vi "Set Tilt Degree (SubVI).vi"(0 "handle in":i64, 1 "degree":i32, 3 "error in (no error)":errorcluster) -> (7 "handle out":i64, 10 "error out":errorcluster)   [LabVIEW 2017]
uses:
  libkinect_wrapper.dll
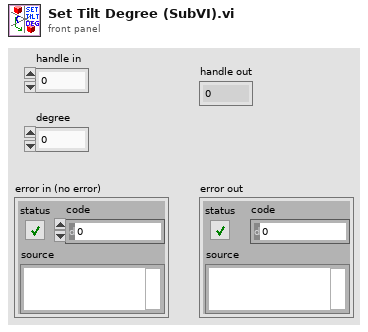
[diagram p1: front panel]
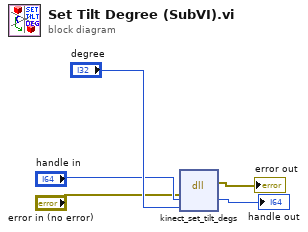
[diagram p0: block diagram]
diagram:
  n1 = dll-call lib="libkinect_wrapper.*" fn="kinect_set_tilt_degs"(error in="error in (no error)", "handle"="handle in", "degree"="degree") -> (error out=→"error out":errorcluster, "handle"=→"handle out":i64)  [unwired: 4 in, 1 out]
